vi "MainRT.vi"() -> ()   [LabVIEW 2017]
doc: "The myRIO Project template acquires acceleration data from the onboard accelerometer and displays the changes of acceleration values in a waveform chart."
uses:
  TypeDefs/CommandsRT.ctl
  Projekt-RubikLibrary/ServoEnumControl.ctl
  Projekt-RubikLibrary/ServoCCWControl.ctl
  TypeDefs/ServoTurnGripCluster.ctl
  <extravilib>/ChannelInstances/Stream-t'DataStreamCluster.ctl'/Read With Abort.vi
  <extravilib>/ChannelInstances/Stream-t'DataStreamCluster.ctl'/Write With Abort.vi
  <vilib>/myRIO/Common/Instrument Driver Framework/myRIO v1.0/UART/vis/myRIO v1.0 Close UART.vi
  <extravilib>/ChannelInstances/Stream-t'DataStreamCluster.ctl'/EndpointRead.vi
  <extravilib>/ChannelInstances/Stream-t'DataStreamCluster.ctl'/Endpoint.vi
  <extravilib>/ChannelInstances/Stream-t'DataStreamCluster.ctl'/Instantiate.vi
  <extravilib>/ChannelInstances/Stream-t'DataStreamCluster.ctl'/)Channel.vi
  <resource>/ChannelSupport/_ChannelSupport/WaitIfNeeded.vi
  <vilib>/myRIO/Common/Instrument Driver Framework/Utilities/vis/FPGA Ref Manager.vi
  <vilib>/myRIO/Common/Instrument Driver Framework/myRIO v1.0/myRIO v1.0 Reset FPGA.vi
  <vilib>/myRIO/Common/Instrument Driver Framework/myRIO v1.0/IRQ/vis/myRIO v1.0 IRQ Info FGV.vi
  <vilib>/myRIO/Common/Instrument Driver Framework/myRIO v1.0/IRQ/vis/myRIO v1.0 Timer IRQ Info FGV.vi
  <vilib>/myRIO/Common/Instrument Driver Framework/myRIO v1.0/IRQ/vis/myRIO v1.0 ISR Agent.vi
  <vilib>/myRIO/Instrument Drivers/Utilities/Utilities.lvlib
  <extravilib>/ChannelInstances/Stream-t'DataStreamCluster.ctl'.lvlib
  Projekt-RubikLibrary/RubikLibrary.lvlib
  Projekt-RubikLibrary/RubikLibraryRT.lvlib
panel:
  out "Turn ccw/cw":T1=enum."ccw"
  out "Servo":T2
  out "State":T3
  out "error out":errorcluster
  # "Overview  MainRT\n\nMainRT on myRIO receives commands from PC via Network Streams.\nMainPC sends commands"
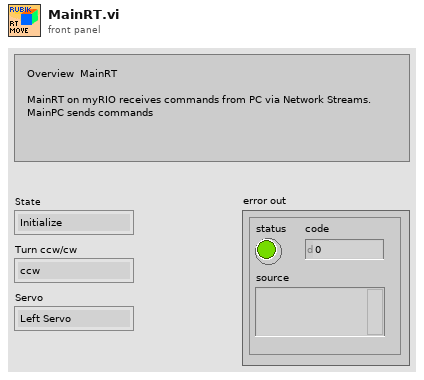
[diagram p1: front panel]
types:
  T1 = typedef "RubikLibrary.lvlib/ServoCCWControl.ctl" = enum16{"cw", "ccw"}
  T2 = typedef "RubikLibrary.lvlib/ServoEnumControl.ctl" = enum16{"Left Servo", "Front Servo", "Right Servo"}
  T3 = typedef "CommandsRT.ctl" = enum16{"Initialize", "Turn", "Grip", "Exit"}
  T4 = typedef "DataStreamCluster.ctl" = cluster{"Commands":T3, "Variant":variant}
  T5 = typedef "Stream-t'DataStreamCluster.ctl'.lvlib/)Channel.ctl" = refnum<queue>
  T6 = typedef "ServoTurnGripCluster.ctl" = cluster{"Servo Enum":T2, "Ang":T1, "Grip":bool}
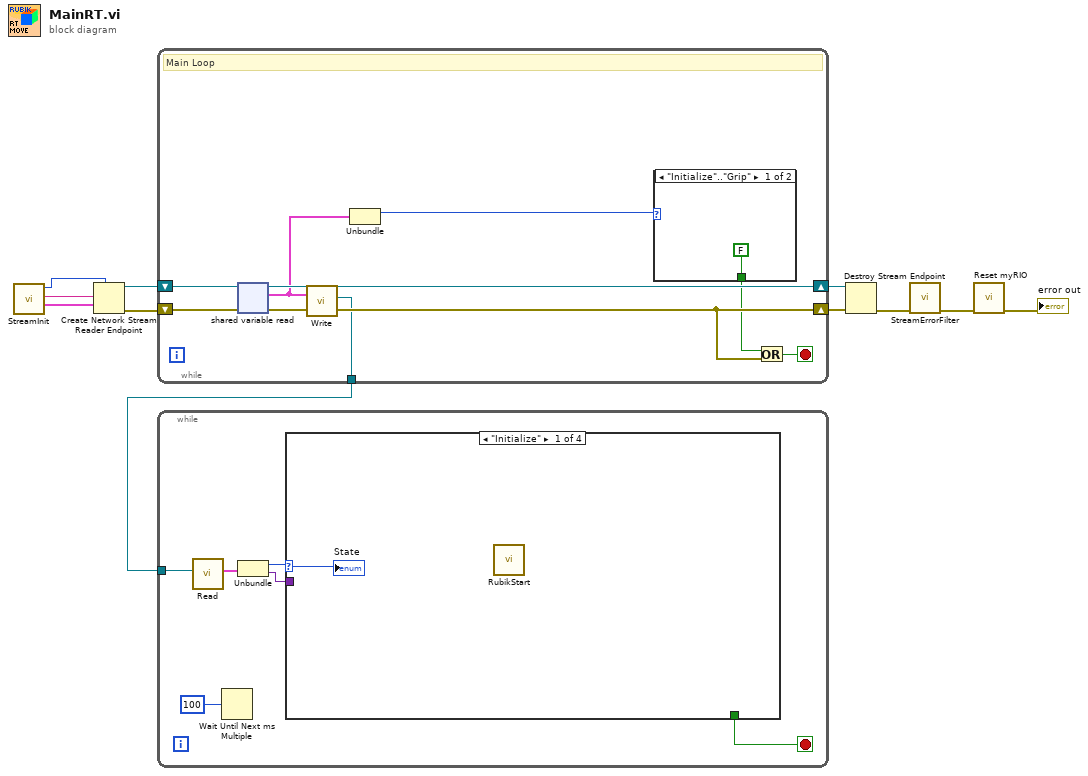
[diagram p0: block diagram]
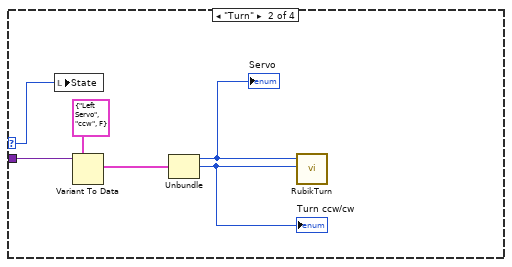
[diagram p2: hidden frame]
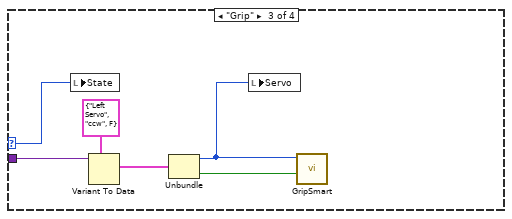
[diagram p3: hidden frame]
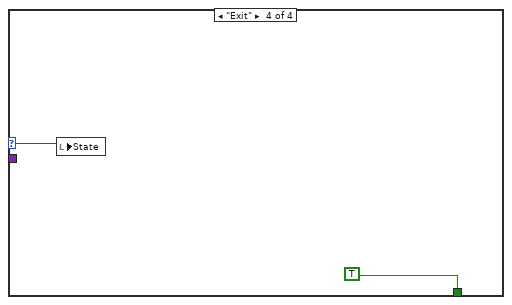
[diagram p4: hidden frame]
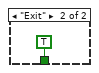
[diagram p5: hidden frame]
diagram:
  n1 = call "StreamInit.vi"() -> ("data cluster"=w3:T4, "reader name"=w2:string, "writer&reader buffer size"=w1:i32)  [unwired: 4 in, 1 out]
  n2 = Create Network Stream Reader Endpoint(7:w1, 9:w3, 11:w2) -> (0:w11:errorcluster, 3:w10:refnum<k21>)  [unwired: 4 in]
  n3 = while {
    shift-right: [w18] -> w7
    shift-left: w11 -> [w18]
    shift-right: [w16] -> w8
    shift-left: w10 -> [w17]
    tunnel: [w14] -> w4
    stop <- w19 stop-if-true
    # "Main Loop"
    n4 = shared-variable-read(w17) -> (w16:refnum<k21>, w13:T4)  [unwired: 2 in, 2 out]
    n5 = call <extravilib>:"Write.vi"("element"=w13) -> ("channel"=w14:T5)  [unwired: 8 in, 2 out]
    n6 = Unbundle(w13) -> ("Commands"=w12:T3)  [unwired: 1 out]
    n7 = case shown="\"Initialize\"..\"Grip\"" w12 {
      tunnel: [FALSE TRUE] -> w15
      frame "Initialize".."Grip" {
      }
      frame "Exit" {
      }
    }
    n8 = Or(x=w15, y=w18) -> (x .or. y?=w19:bool)
  }
  n9 = while {
    tunnel: w4 -> [w25]
    stop <- w27 stop-if-true
    n10 = call <extravilib>:"Read.vi"("channel"=w25) -> ("element"=w24:T4)  [unwired: 6 in, 4 out]
    n11 = Wait Until Next ms Multiple(millisecond multiple=u32 100) -> ()  [unwired: 1 out]
    n12 = Unbundle(w24) -> ("Commands"=w23:T3, "Variant"=w22:variant)
    n13 = case shown="\"Initialize\"" w23 {
      selector: w23 -> [w28 w34 w40 w41]
      tunnel: [_ _ _ TRUE] -> w27
      tunnel: w22 -> [_ w33 w39 _]
      frame "Initialize" {
        n14 = call "RubikStart.vi"() -> ()  [unwired: 11 in, 1 out]
        "State" <- w28
      }
      frame "Turn" {
        n15 = local write "State"(w34) -> ()
        n16 = Variant To Data(type=T6 {"Servo Enum"=enum."Left Servo", "Ang"=enum."ccw", "Grip"=FALSE} ("Cluster:  Servo to turn and grip"), Variant=w33) -> (data=w31:T6)  [unwired: 1 in, 1 out]
        n17 = Unbundle(w31) -> ("Servo Enum"=w32:T2, "Ang"=w29:T1)  [unwired: 1 out]
        "Servo" <- w32
        "Turn ccw/cw" <- w29
        n18 = call "RubikTurn.vi"("Turn"=w29, "Servo"=w32) -> ()  [unwired: 2 in, 2 out]
      }
      frame "Grip" {
        # "Nothing to do"
        n19 = local write "State"(w40) -> ()
        n20 = Variant To Data(type=T6 {"Servo Enum"=enum."Left Servo", "Ang"=enum."ccw", "Grip"=FALSE} ("Cluster:  Servo to turn and grip"), Variant=w39) -> (data=w37:T6)  [unwired: 1 in, 1 out]
        n21 = Unbundle(w37) -> ("Servo Enum"=w38:T2, "Grip"=w36:bool)  [unwired: 1 out]
        n22 = local write "Servo"(w38) -> ()
        n23 = call "GripSmart.vi"("Grip closed (in)"=w36, "Servo"=w38) -> ()  [unwired: 8 in, 2 out]
      }
      frame "Exit" {
        n24 = local write "State"(w41) -> ()
      }
    }
  }
  n25 = Destroy Stream Endpoint(8:w7, 11:w8) -> (0:w9:errorcluster)
  n26 = call "StreamErrorFilter.vi"("error in (no error)"=w9) -> ("error out"=w5:errorcluster)  [unwired: 10 in]
  n27 = call <vilib>:"Reset myRIO.vi"("error in (no error)"=w5) -> ("error out"=→"error out":errorcluster)  [unwired: 10 in]
